vi "Update Parameter Data Pointers.vi"(7 "Data Pointer":u16 format="%04x", 8 "error in (no error)":errorcluster, 11 "Filter in":refnum<class "Filter.lvclass">) -> (0 "error out":errorcluster, 3 "Filter out":refnum<class "Filter.lvclass">)   [LabVIEW 2020, in "BCI-1553 API.lvlib" / "Filter.lvclass"]
doc: "<DO NOT CALL>\n\nThis method is leveraged by the Bus Monitor to properly track parameters in a Bus Monitor application."
uses:
  Filter.lvclass
  Filter.lvclass/Filter.ctl
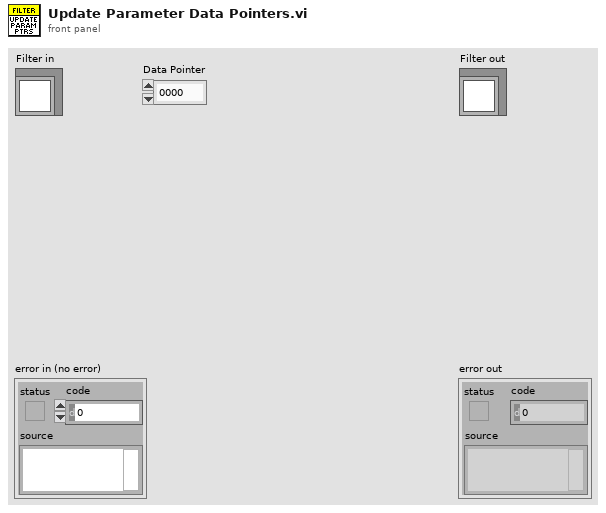
[diagram p1: front panel]
types:
  T1 = typedef "BCI-1553 API.lvlib/Parameter Table Data.ctl" = cluster{"Parameter Name":string, "Base Word":u16, "Address":u16, "Value":u64, "Mask":u16[], "Scaling Info":T2}
  T2 = typedef "BCI-1553 API.lvlib/Scaling Information.ctl" = cluster{"Bit Offset":i32, "Bit Count":i32, "LSB Resolution":dbl, "2's Complement":bool, "Big Endian":bool, "Sign Bit":bool}
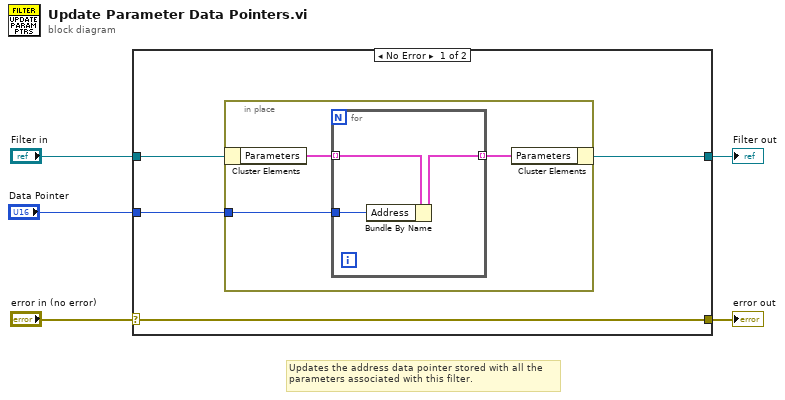
[diagram p0: block diagram]
diagram:
  # "Updates the address data pointer stored with all the\nparameters associated with this filter."
  n1 = case shown="No Error" "error in (no error)" {
    selector: "error in (no error)" -> [w9 w17]
    tunnel: [w9 w17] -> w4
    tunnel: [w7 w16] -> w2
    tunnel: "Filter in" -> [w8 w16]
    tunnel: "Data Pointer" -> [w6 _]
    frame No Error {
      n2 = in-place {
        in-place-border: w6 -> [w10]
        n3 = in-place-cluster #1(w8) -> ("Parameters"=w12:T1[])
        n4 = for {
          tunnel: w12 -> [w15] mode=indexing
          tunnel: [w14] -> w11 mode=indexing
          tunnel: w10 -> [w13]
          n5 = Bundle By Name(cluster=w15, "Address"=w13) -> (w14:T1)
        }
        n6 = in-place-cluster #1("Parameters"=w11) -> (w7:refnum<class "Filter.lvclass">)
      }
    }
    frame Error {
    }
  }
  "error out" <- w4
  "Filter out" <- w2
